vi "DB_Global.vi"() -> ()   [LabVIEW 2025]
uses:
  <vilib>/ActorFramework/Message Enqueuer/Message Enqueuer.lvclass
panel:
  in  "Database":refnum<class "Message Enqueuer.lvclass">
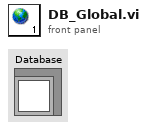
[diagram p1: front panel]
diagram:
